vi "Digital IO Message - Continuous Port Report.vi"(8 "error in (no error)":errorcluster, 9 "Enable Continuous Reporting?":bool, 10 "Port Index":u8 format="%x") -> (0 "error out":errorcluster, 1 "PortValue":u16, 2 "Port Index Out":u8, 4 "PortValueAsArray":bool[](array[boolean]))   [LabVIEW 2020, in "FirmataClient.lvlib"]
doc: "Allows requesting the state of a digital port."
uses:
  FirmataClient.lvlib
panel:
  in  "Queue Name":string="firmata-serial-communication"
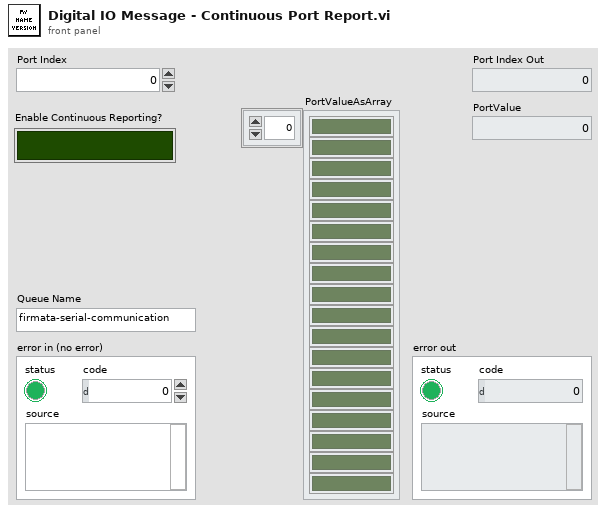
[diagram p1: front panel]
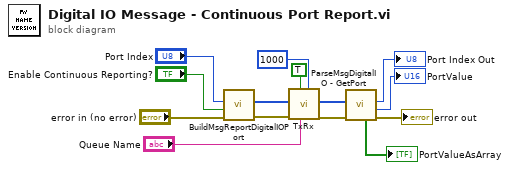
[diagram p0: block diagram]
diagram:
  n1 = call "BuildMsgReportDigitalIOPort.vi"("error in"="error in (no error)", "Enable Continuous Reporting?"="Enable Continuous Reporting?", "Port Index"="Port Index") -> ("error out"=w4:errorcluster, "DigitalIOMessage"=w3:u8[])  [unwired: 5 in, 2 out]
  n2 = call "TxRx.vi"("Reply Timeout Ms"=1000, "Queue Name"="Queue Name", "Wait For Reply?"=TRUE, "error in"=w4, "Message"=w3) -> ("error out"=w1:errorcluster, "Reply"=w2:u8[])  [unwired: 5 in]
  n3 = call "ParseMsgDigitalIO - GetPort.vi"("error in"=w1, "Message"=w2) -> ("error out"=→"error out":errorcluster, "PortValue"=→"PortValue":u16, "Port Index"=→"Port Index Out":u8, "PortValueAsArray"=→"PortValueAsArray":bool[])  [unwired: 6 in]
